vi "Min_VI.vi"() -> ()   [LabVIEW 2018]
panel:
  out "y":dbl
  in  "b":dbl
  in  "a":dbl
  in  "x":dbl
  in  "stop":bool
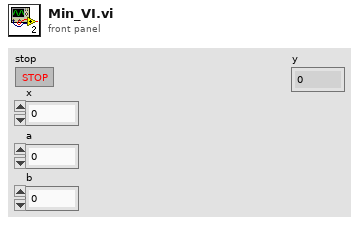
[diagram p1: front panel]
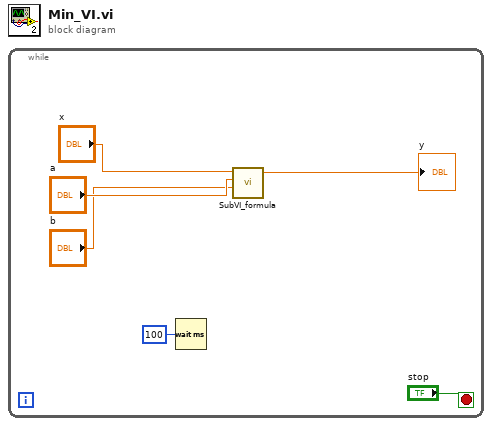
[diagram p0: block diagram]
diagram:
  n1 = while {
    stop <- "stop" stop-if-true
    n2 = Wait (ms)(milliseconds to wait=u32 100) -> ()  [unwired: 1 out]
    n3 = call "SubVI_formula.vi"("b"="b", "a"="a", "x"="x") -> ("y"=→"y":dbl)  [unwired: 8 in]
  }
